vi "Actor Core.vi"(8 "error in":errorcluster, 11 "View in":refnum<class "RTM List View.lvclass">) -> (0 "error out":errorcluster, 3 "Actor out":refnum<class "Actor.lvclass">)   [LabVIEW 2013, in "SET Project Editor.lvlib" / "RTM List View.lvclass"]
doc: "(<B>Filename</B>: Actor Framework.lvlib:Actor.lvclass:Actor Core.vi)\n\nReceives messages to the actor, reacts to them, and initiates any error handling that may shut the actor down.\n\nDescendant classes may override this VI to append parallel tasks for the actor to complete while it handles messages. Overrides use the Call Parent Method node."
uses:
  RTM List View.lvclass
  <vilib>/ActorFramework/Actor/Actor.lvclass
  <vilib>/ActorFramework/Actor/Actor.lvclass/Actor.ctl
  <vilib>/ActorFramework/Message Enqueuer/Message Enqueuer.lvclass/Message Enqueuer.ctl
  Controller Messages/Change Selection Msg/Change Selection Msg.lvclass/Change Selection Msg.ctl
  Controller Messages/Remove Object Msg/Remove Object Msg.lvclass/Remove Object Msg.ctl
  RTM List View.lvclass/RTM List View.ctl
  UI View/UI View.lvclass
  <vilib>/ActorFramework/Message Enqueuer/Init from Existing Queue.vi
  <vilib>/ActorFramework/Message Enqueuer/Enqueue.vi
  <vilib>/ActorFramework/Message Priority Queue/Priority Enqueue.vi
  <vilib>/ActorFramework/Message Enqueuer/Message Enqueuer.lvclass
  <vilib>/ActorFramework/Stop Msg/Stop Msg.lvclass
  Controller Messages/Change Selection Msg/Change Selection Msg.lvclass
  Controller Messages/Remove Object Msg/Remove Object Msg.lvclass
panel:
  in  "Items":i32(listbox)
  # "Run-Time Menu List"
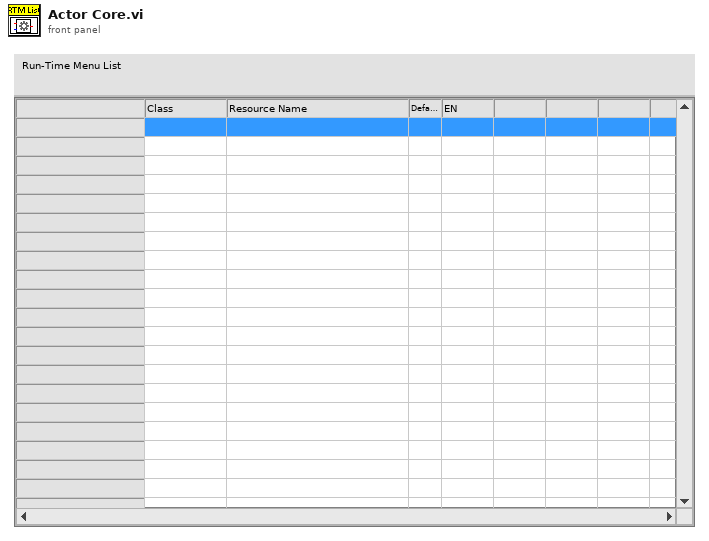
[diagram p1: front panel]
types:
  T1 = typedef "LVPoint32TypeDef.ctl" = cluster{"Horizontal":i32, "Vertical":i32}
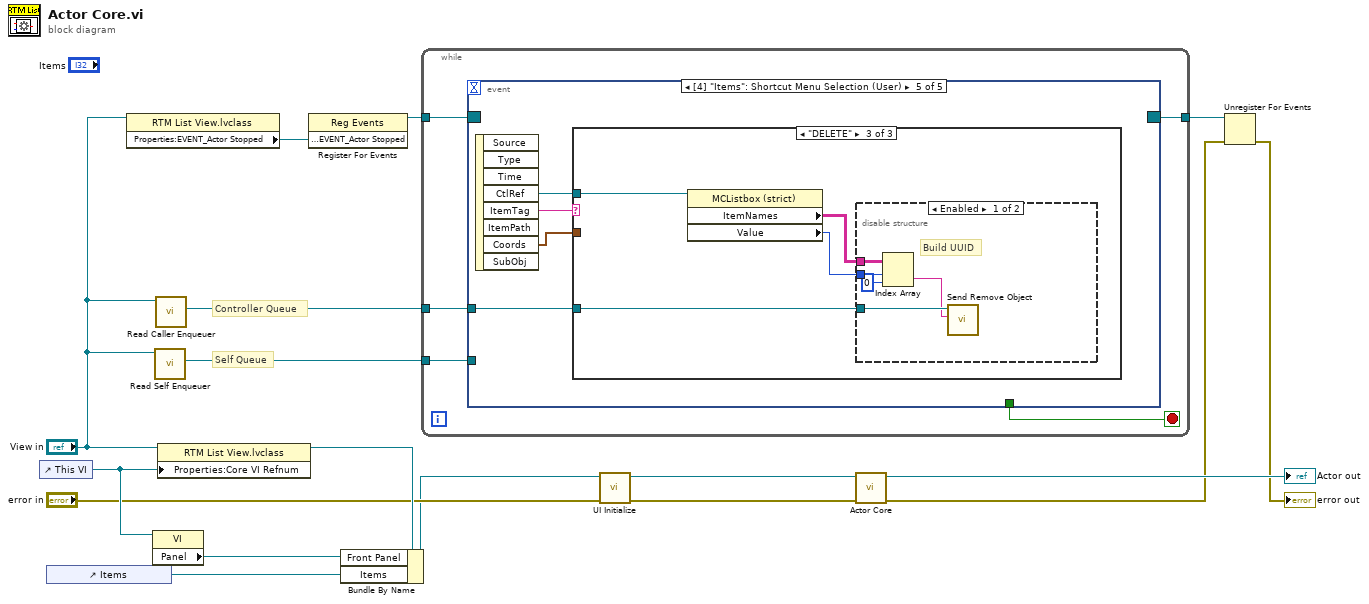
[diagram p0: block diagram]
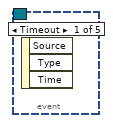
[diagram p2: hidden frame]
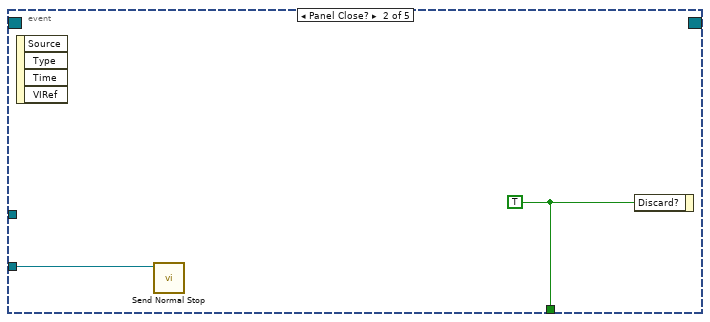
[diagram p3: hidden frame]
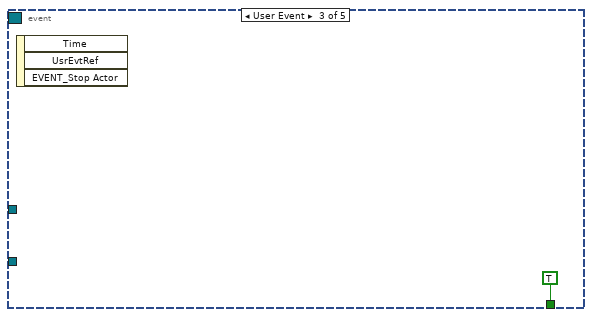
[diagram p4: hidden frame]
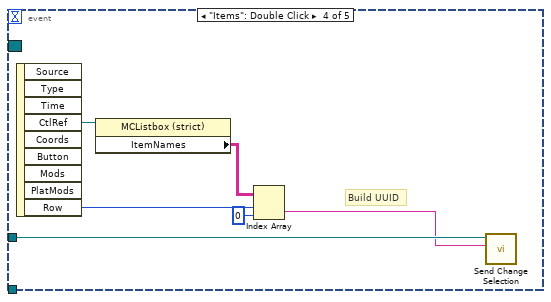
[diagram p5: hidden frame]
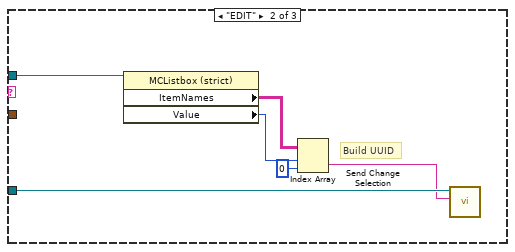
[diagram p7: hidden frame]
diagram:
  # "Controller Queue"
  # "Self Queue"
  n1 = control-ref of="This VI"() -> (w8:refnum<vi>)
  n2 = control-ref of="Items"() -> (w6:refnum<vi>)
  n3 = property class="RTM List View.lvclass"(reference="View in") -> ("Properties:EVENT_Actor Stopped"=w16:refnum<user-event>)  [unwired: 1 in, 2 out]
  n4 = property class="VI"(reference=w8) -> ("Panel"=w7:refnum<vi>)  [unwired: 1 in, 2 out]
  n5 = call <vilib>:"Read Self Enqueuer.vi"("Actor"="View in") -> ("Self Enqueuer"=w5:refnum<class "Message Enqueuer.lvclass">)  [unwired: 10 in]
  n6 = call <vilib>:"Read Caller Enqueuer.vi"("Actor"="View in") -> ("Caller Enqueuer"=w11:refnum<class "Message Enqueuer.lvclass">)  [unwired: 10 in]
  n7 = property class="RTM List View.lvclass"(reference="View in", "Properties:Core VI Refnum"=w8) -> (reference out=w9:refnum<class "RTM List View.lvclass">)  [unwired: 1 in, 1 out]
  n8 = register-events(w16) -> (reference out=w15:refnum<event-registration>)  [unwired: 2 in, 1 out]
  n9 = Bundle By Name(cluster=w9, "Front Panel"=w7, "Items"=w6) -> (w1:refnum<class "RTM List View.lvclass">)
  n10 = while {
    tunnel: w15 -> [w21]
    tunnel: [w20] -> w14
    tunnel: w5 -> [w19]
    tunnel: w11 -> [w18]
    stop <- w22 stop-if-true
    n11 = event shown="[4] \"Items\": Shortcut Menu Selection (User)" {
      selector: w21 -> [_ _ _ _ _]
      dyn-events: [_ _ _ _ _] -> w20
      timeout: _ -> [_ _ _ _ _]
      tunnel: [_ w24 TRUE ("Discard?") _ _] -> w22
      tunnel: w19 -> [_ w23 _ _ _]
      tunnel: w18 -> [_ _ _ w28 w32]
      event Timeout {
        n12 = event-data() -> ()  [unwired: 1 in, 3 out]
      }
      event Panel Close? {
        w24 = TRUE ("Discard?")
        n13 = event-data() -> ()  [unwired: 1 in, 4 out]
        n14 = call <vilib>:"Send Normal Stop.vi"("Message Enqueuer"=w23) -> ()  [unwired: 10 in, 1 out]
        n15 = event-data("Discard?"=w24) -> ()  [unwired: 1 in, 1 out]
      }
      event User Event {
        n16 = event-data() -> ()  [unwired: 1 in, 3 out]
      }
      event "Items": Double Click {
        # "Build UUID"
        n17 = event-data() -> ("CtlRef"=w31:refnum<vi>, "Row"=w29:i32)  [unwired: 1 in, 7 out]
        n18 = property class="MCListbox (strict)"(reference=w31) -> ("ItemNames"=w30:string[][])  [unwired: 1 in, 2 out]
        n19 = Index Array(array=w30, index (row)=w29, index (col)=0 ("disabled index (col)")) -> (element=w27:string)
        n20 = call "Send Change Selection.vi"("UID"=w27, "Message Enqueuer"=w28) -> ()  [unwired: 8 in, 2 out]
      }
      event "Items": Shortcut Menu Selection (User) {
        n21 = event-data() -> ("CtlRef"=w34:refnum<vi>, "ItemTag"=w35:string, "Coords"=w33:T1)  [unwired: 1 in, 5 out]
        n22 = case shown="\"DELETE\"" w35 {
          tunnel: w34 -> [_ w39 w43]
          tunnel: w33 -> [_ _ _]
          tunnel: w32 -> [_ w38 w42]
          frame Default {
          }
          frame "EDIT" {
            # "Build UUID"
            n23 = property class="MCListbox (strict)"(reference=w39) -> ("ItemNames"=w40:string[][], "Value"=w41:i32)  [unwired: 1 in, 2 out]
            n24 = Index Array(array=w40, index (row)=w41, index (col)=0 ("disabled index (col)")) -> (element=w36:string)
            n25 = call "Send Change Selection.vi"("UID"=w36, "Message Enqueuer"=w38) -> ()  [unwired: 8 in, 2 out]
          }
          frame "DELETE" {
            n26 = property class="MCListbox (strict)"(reference=w43) -> ("ItemNames"=w44:string[][], "Value"=w45:i32)  [unwired: 1 in, 2 out]
            n27 = disable-structure shown="Enabled" {
              disable-tunnel: w45 -> [w50 _]
              disable-tunnel: w44 -> [w49 _]
              disable-tunnel: w42 -> [w47 _]
              frame Enabled {
                # "Build UUID"
                n28 = Index Array(array=w49, index (row)=w50, index (col)=0 ("disabled index (col)")) -> (element=w46:string)
                n29 = call "Send Remove Object.vi"("UUID"=w46, "Message Enqueuer"=w47) -> ()  [unwired: 8 in, 2 out]
              }
              frame Disabled {
              }
            }
          }
        }
      }
    }
  }
  n30 = call-dynamic "UI Initialize.vi"("error in (no error)"="error in", "GObject View in"=w1) -> ("error out"=w3:errorcluster, "GObject View out"=w4:refnum<class "RTM List View.lvclass">)  [unwired: 8 in]
  n31 = call-parent "Actor Core.vi"("error in"=w3, "Actor in"=w4) -> ("error out"=w13:errorcluster, "Actor out"=→"Actor out":refnum<class "Actor.lvclass">)  [unwired: 8 in]
  n32 = Unregister For Events(event registration refnum=w14, error in=w13) -> (error out=→"error out":errorcluster)
